vi "Apply Hardware Configurations.vi"(8 "error in (no error)":errorcluster, 9 "HW Config Object":refnum<class "HW Configuration.lvclass">, 10 "Device Name":string, 11 "Controller in":refnum<class "Controller.lvclass">) -> (0 "error out":errorcluster, 3 "Controller out":refnum<class "Controller.lvclass">)   [LabVIEW 2017, in "Controller Actor.lvlib" / "Controller.lvclass"]
uses:
  Controller.lvclass
  Hardware/HW Config/HW Configuration.lvclass
  Hardware/Hardware.lvclass
  Controller.lvclass/Controller.ctl
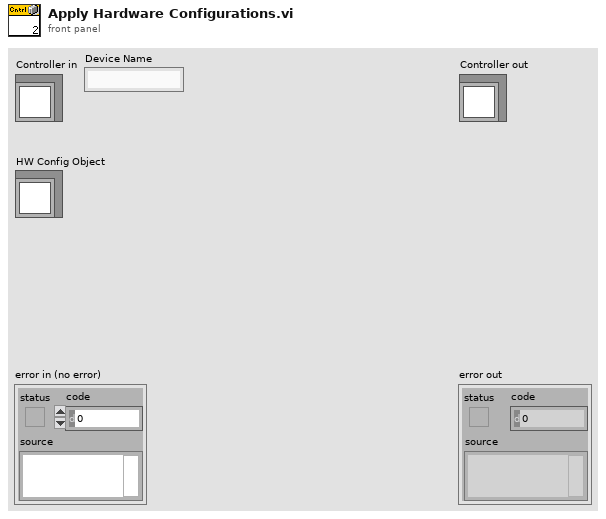
[diagram p1: front panel]
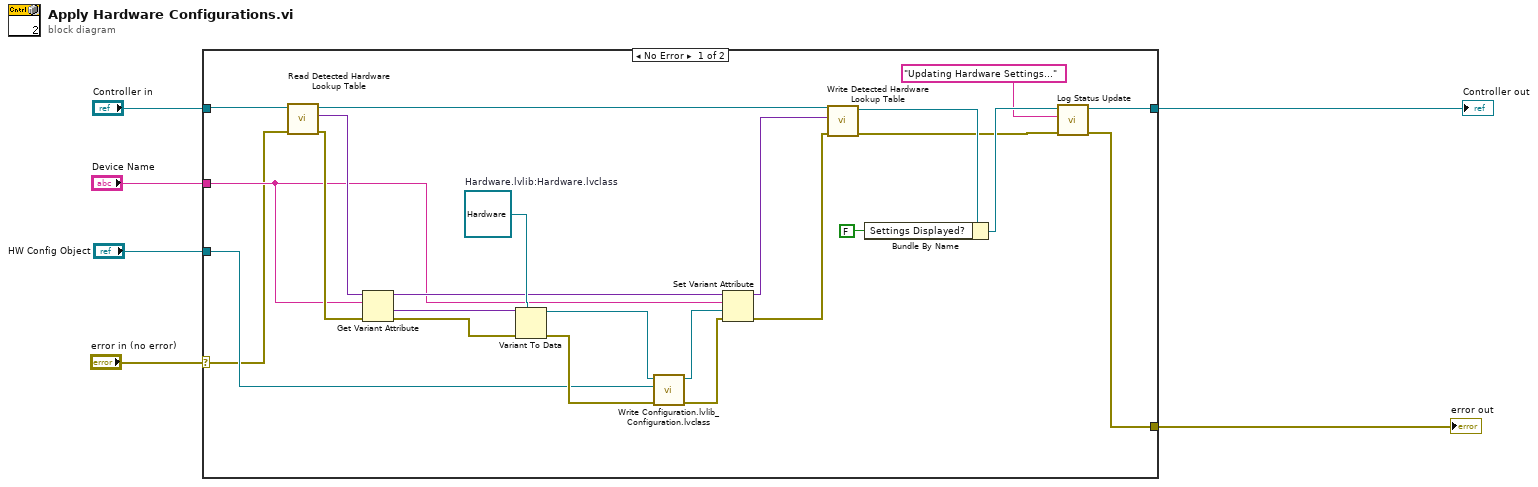
[diagram p0: block diagram]
diagram:
  n1 = case shown="No Error" "error in (no error)" {
    selector: "error in (no error)" -> [w12 w32]
    tunnel: [w8 w32] -> w5
    tunnel: [w10 w31] -> w3
    tunnel: "Controller in" -> [w16 w31]
    tunnel: "HW Config Object" -> [w14 _]
    tunnel: "Device Name" -> [w13 _]
    frame No Error {
      w27 = refnum<class "Hardware.lvclass"> refnum  # Hardware.lvlib:Hardware.lvclass
      n2 = call "Read Detected Hardware Lookup Table.vi"("error in (no error)"=w12, "Controller in"=w16) -> ("error out"=w29:errorcluster, "Detected Hardware Lookup Table"=w30:variant, "Controller out"=w15:refnum<class "Controller.lvclass">)  [unwired: 7 in]
      n3 = Get Variant Attribute(Variant=w30, name=w13, error in=w29) -> (duplicate Variant=w23:variant, value=w28:variant, error out=w26:errorcluster)  [unwired: 1 in, 1 out]
      n4 = Variant To Data(error in=w26, type=w27, Variant=w28) -> (data=w25:refnum<class "Hardware.lvclass">, error out=w21:errorcluster)
      n5 = call-dynamic "Write Configuration.lvlib_Configuration.lvclass.vi"("error in (no error)"=w21, "Hardware.lvlib:HW Configuration.lvclass"=w14, "Hardware in"=w25) -> ("error out"=w22:errorcluster, "Hardware out"=w24:refnum<class "Hardware.lvclass">)  [unwired: 7 in]
      n6 = Set Variant Attribute(Variant=w23, name=w13, value=w24, error in=w22) -> (Variant out=w20:variant, error out=w17:errorcluster)  [unwired: 1 out]
      n7 = call "Write Detected Hardware Lookup Table.vi"("error in (no error)"=w17, "Detected Hardware Lookup Table"=w20, "Controller in"=w15) -> ("error out"=w9:errorcluster, "Controller out"=w19:refnum<class "Controller.lvclass">)  [unwired: 7 in]
      n8 = Bundle By Name(cluster=w19, "Settings Displayed?"=FALSE) -> (w11:refnum<class "Controller.lvclass">)
      n9 = call-dynamic "Log Status Update.vi"("error in (no error)"=w9, "String"="Updating Hardware Settings...", "Controller in"=w11) -> ("error out"=w8:errorcluster, "Controller out"=w10:refnum<class "Controller.lvclass">)  [unwired: 7 in]
    }
    frame Error {
    }
  }
  "error out" <- w5
  "Controller out" <- w3
